vi "Main.vi"() -> ()   [LabVIEW 2019]
uses:
  _Sound/Music Player Command Message.ctl
  _Sound/Music Player Command.ctl
  <vilib>/numeric/Random Number (Range) DBL.vi
  <vilib>/numeric/Random Number (Range) U64.vi
  <vilib>/numeric/sub_Random U32.vi
  _Sound/Sound.lvlib
panel:
  in  "Enable Disasters":bool
  in  "Disaster Ring":u16(ring) caption="Disaster" items=["Earthquake", "Tornado", "UFO", "» Apocalypse «"]
  in  "Launch Disaster":bool
  in  "Enable Sounds":bool=TRUE
  in  "Random":bool
  out "Now Playing::":string
  in  "Enable Music":bool=TRUE
  in  "Random Disasters":bool
  out "LED Yellow Left":bool[](array[boolean])
  out "LED Yellow Right":bool[](array[boolean])
  out "LED Yellow Bottom":bool[](array[boolean])
  out "LED Yellow Top":bool[](array[boolean])
  out "LED Red Top":bool[](array[boolean])
  out "LED Red Right":bool[](array[boolean])
  out "LED Red Bottom":bool[](array[boolean])
  out "LED Red Left":bool[](array[boolean])
  out "Disasters":bool
  # "SimCity 2000\nToolkit for LabVIEW"
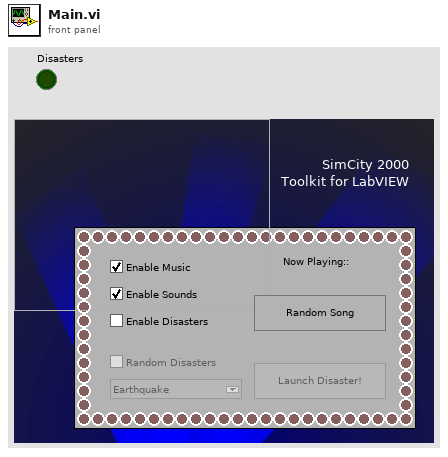
[diagram p1: front panel]
types:
  T1 = enum8{"Enabled", "Disabled", "Disabled and Grayed Out"}
  T2 = typedef "Sound.lvlib/Music Player Command Message.ctl" = cluster{"Command":T3, "Data":variant}
  T3 = typedef "Sound.lvlib/Music Player Command.ctl" = enum16{"Enable", "Play", "Play Random", "Stop", "Shutdown"}
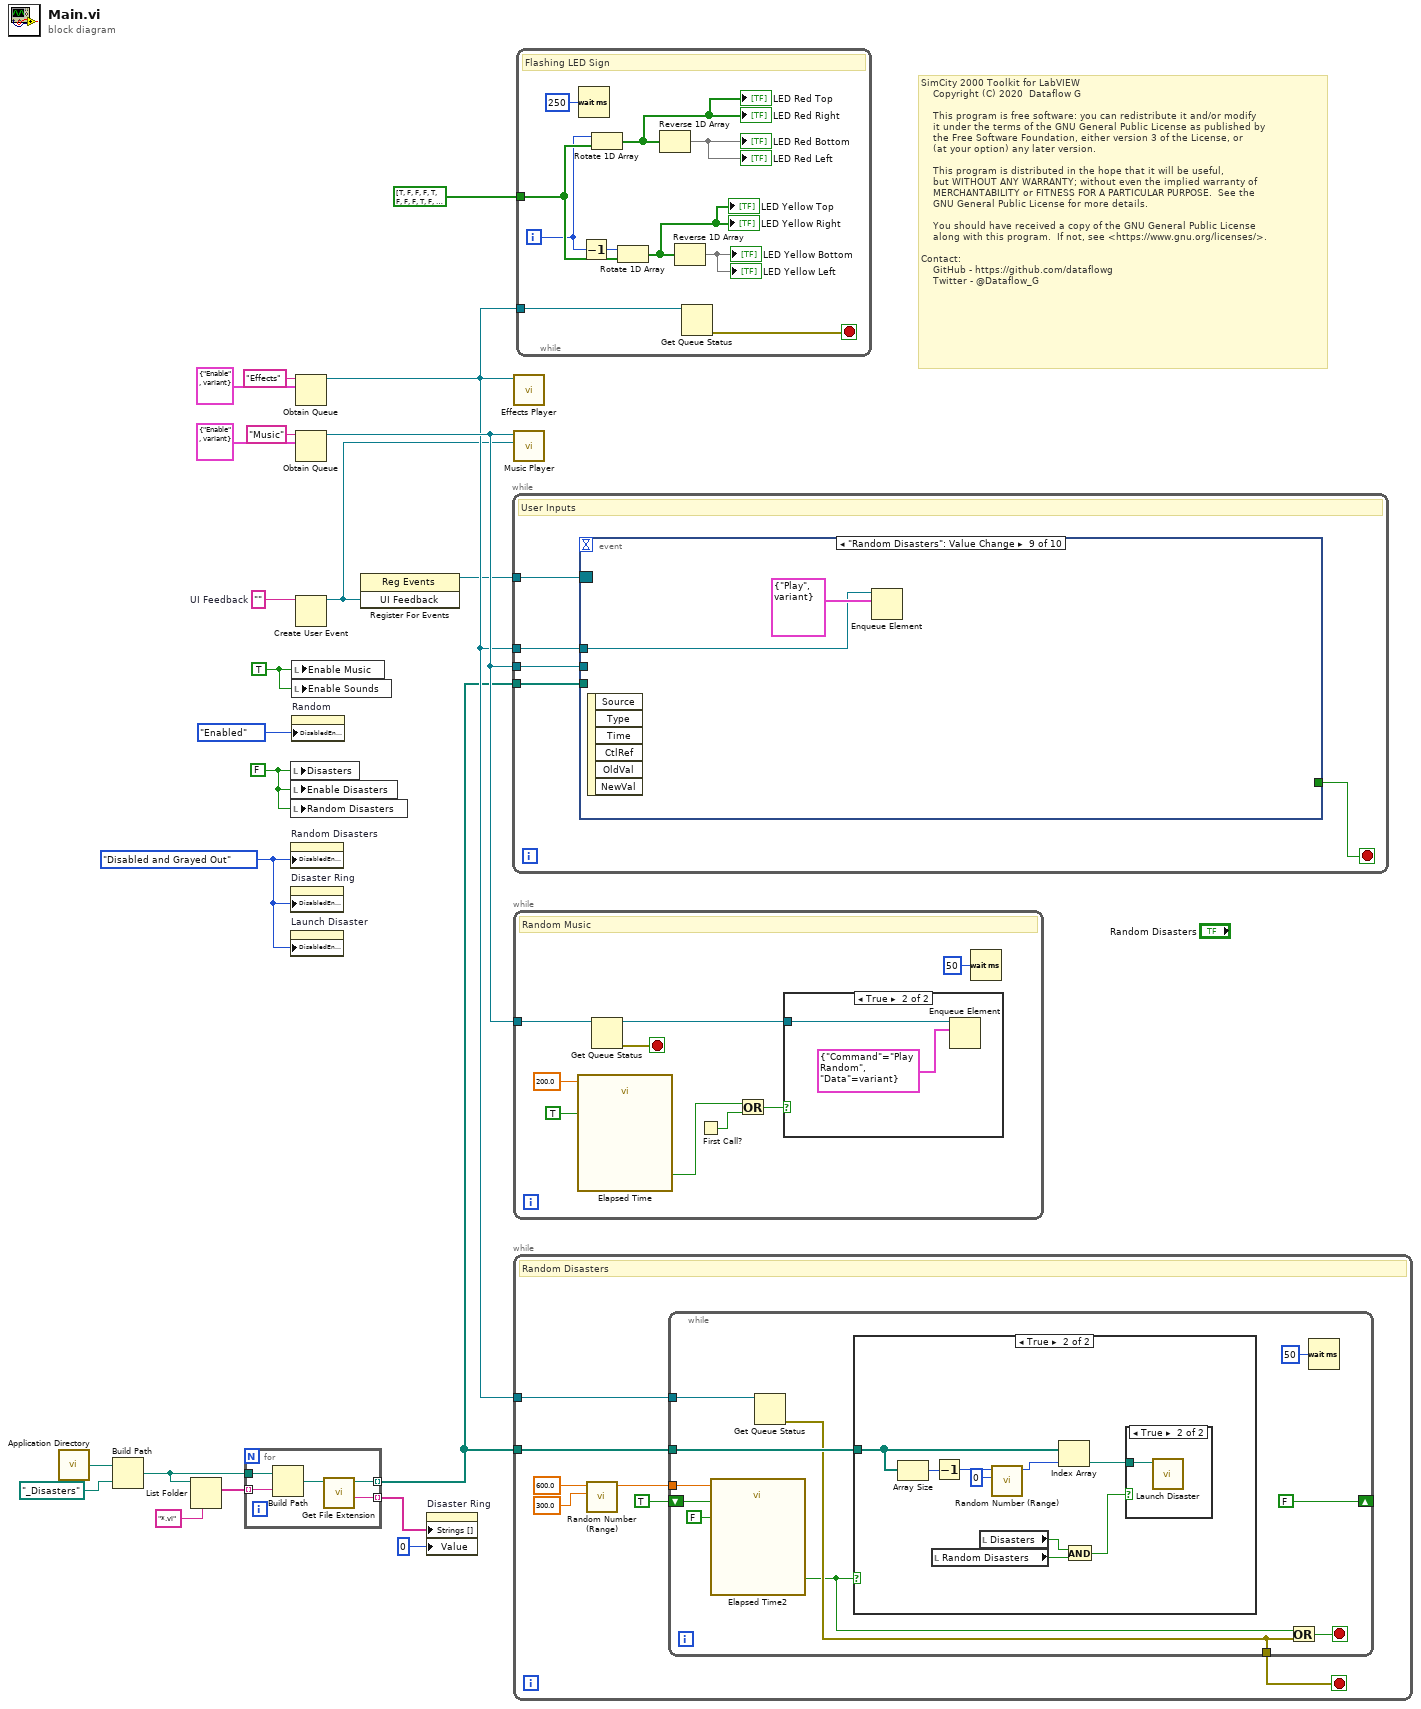
[diagram p0: block diagram]
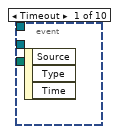
[diagram p5: hidden frame]
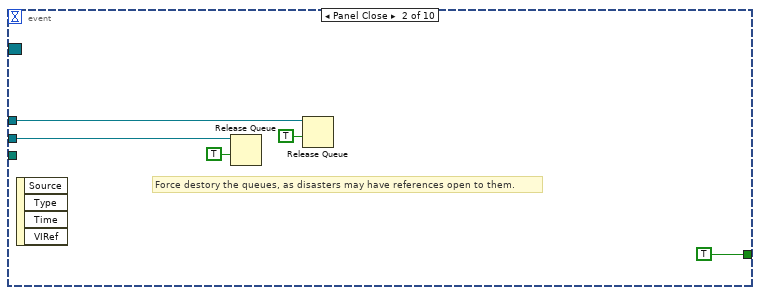
[diagram p6: hidden frame]
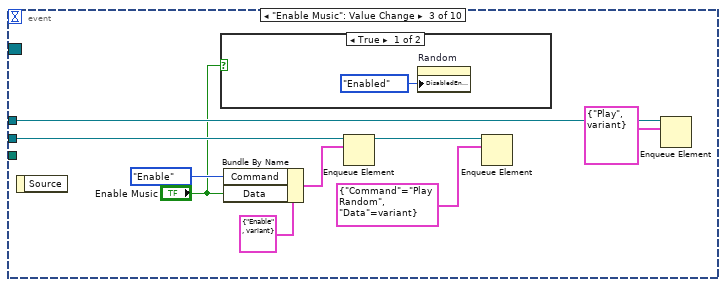
[diagram p7: hidden frame]
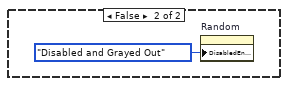
[diagram p8: hidden frame]
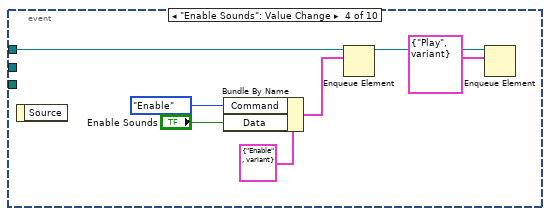
[diagram p9: hidden frame]
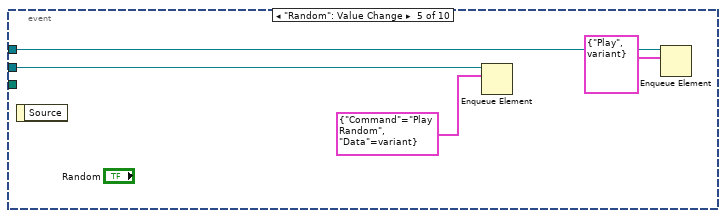
[diagram p10: hidden frame]
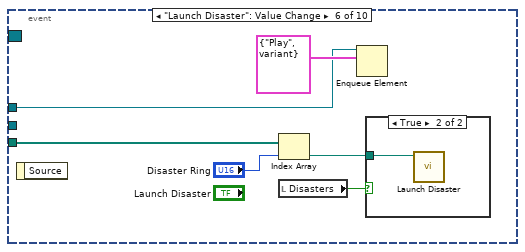
[diagram p11: hidden frame]
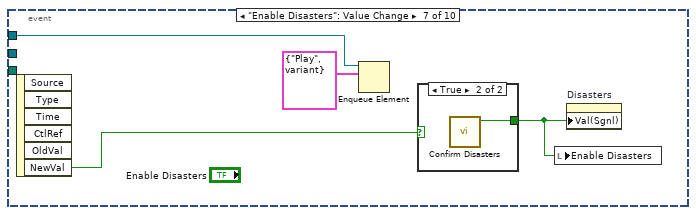
[diagram p13: hidden frame]
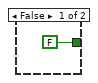
[diagram p14: hidden frame]
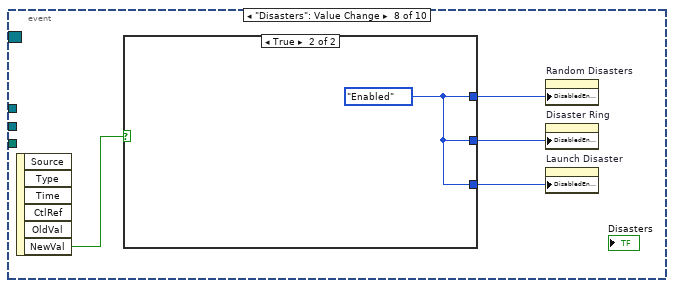
[diagram p15: hidden frame]
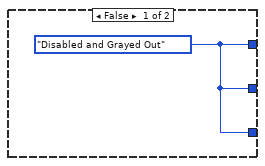
[diagram p16: hidden frame]
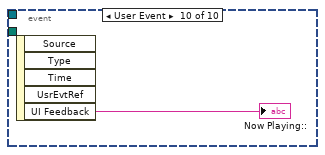
[diagram p17: hidden frame]
diagram:
  w1 = FALSE ("Disasters")
  w2 = TRUE ("Enable Music")
  w4 = T1."Disabled and Grayed Out" ("Disabled")
  w13 = ""  # UI Feedback
  # "SimCity 2000 Toolkit for LabVIEW\n    Copyright (C) 2020  Dataflow G\n    \n    This program is free software: you can redistribute it and/or modify\n    it under the terms of the GNU General Public License as published by\n    the Free Software Foundation, either version 3 of the License, or\n    (at your option) any later version.\n\n    This program is distributed in the hope that it will be useful,\n    but WITHOUT ANY WARRANTY; without even the implied warranty of\n    MERCHANTABILITY or FITNESS FOR A PARTICULAR PURPOSE.  See the\n    GNU General Public License for more details.\n\n    You should have received a copy of the GNU General Public License\n    along with this program.  If not, see <https://www.gnu.org/licenses/>.\n\nContact:\n    GitHub - https://github.com/dataflowg\n    Twitter - @Dataflow_G"
  n1 = call <vilib>:"Application Directory.vi"() -> ("Application Directory"=w20:path)
  n2 = Build Path(base path=w20, name or relative path=path "_Disasters" ("path")) -> (appended path=w10:path)
  n3 = List Folder(path=w10, pattern="*.vi") -> (filenames=w9:string[])  [unwired: 2 in, 3 out]
  n4 = for {
    tunnel: w10 -> [w27]
    tunnel: w9 -> [w26] mode=indexing
    tunnel: [w24] -> w7 mode=indexing
    tunnel: [w23] -> w5 mode=indexing
    n5 = Build Path(base path=w27, name or relative path=w26) -> (appended path=w25:path)
    n6 = call <vilib>:"Get File Extension.vi"("file"=w25) -> ("filename without extension"=w24:string, "dup file"=w23:path)  [unwired: 6 in, 3 out]
  }
  n7 = local write "Disasters"(w1) -> ()
  n8 = local write "Enable Disasters"(w1) -> ()
  n9 = local write "Random Disasters"(w1) -> ()
  n10 = property on="Random Disasters" class="Bool (strict)"("DisabledEnum"=w4) -> ()  [unwired: 2 in, 2 out]
  n11 = property on="Disaster Ring" class="Ring (strict)"("DisabledEnum"=w4) -> ()  [unwired: 2 in, 2 out]
  n12 = property on="Launch Disaster" class="Bool"("DisabledEnum"=w4) -> ()  [unwired: 2 in, 2 out]
  n13 = local write "Enable Music"(w2) -> ()
  n14 = local write "Enable Sounds"(w2) -> ()
  n15 = property on="Random" class="Bool"("DisabledEnum"=T1."Enabled" ("Disabled")) -> ()  [unwired: 2 in, 2 out]
  n16 = Obtain Queue(name (unnamed)="Effects", element data type=T2 {"Command"=enum."Enable", "Data"=variant} ("Message")) -> (queue out=w16:refnum<queue>)  [unwired: 3 in, 2 out]
  n17 = Obtain Queue(name (unnamed)="Music", element data type=T2 {"Command"=enum."Enable", "Data"=variant} ("Message")) -> (queue out=w19:refnum<queue>)  [unwired: 3 in, 2 out]
  n18 = Create User Event(user event datatype=w13) -> (user event=w12:refnum<user-event>)  [unwired: 1 in, 1 out]
  n19 = register-events(w12) -> (reference out=w11:refnum<event-registration>)  [unwired: 2 in, 1 out]
  n20 = property on="Disaster Ring" class="Ring (strict)"("Strings []"=w7, "Value"=u16 0) -> ()  [unwired: 2 in, 2 out]
  n21 = while {
    tunnel: w19 -> [w32]
    tunnel: w16 -> [w31]
    tunnel: w11 -> [w29]
    tunnel: w5 -> [w28]
    stop <- w30 stop-if-true
    # "User Inputs"
    n22 = event shown="[8] \"Random Disasters\": Value Change" {
      selector: w29 -> [_ _ _ _ _ _ _ _ _ _]
      dyn-events: _ -> [_ _ _ _ _ _ _ _ _ _]
      timeout: _ -> [_ _ _ _ _ _ _ _ _ _]
      tunnel: w32 -> [_ w37 w44 _ w56 _ _ _ _ _]
      tunnel: w31 -> [_ w36 w42 w50 w59 w60 w68 _ w79 _]
      tunnel: [_ TRUE _ _ _ _ _ _ _ _] -> w30
      tunnel: w28 -> [_ _ _ _ _ w65 _ _ _ _]
      event Timeout {
        n23 = event-data() -> ()  [unwired: 1 in, 3 out]
      }
      event Panel Close {
        # "Force destory the queues, as disasters may have references open to them."
        n24 = event-data() -> ()  [unwired: 1 in, 4 out]
        n25 = Release Queue(queue=w37, force destroy? (F)=TRUE) -> ()  [unwired: 1 in, 3 out]
        n26 = Release Queue(queue=w36, force destroy? (F)=TRUE) -> ()  [unwired: 1 in, 3 out]
      }
      event "Enable Music": Value Change {
        n27 = event-data() -> ()  [unwired: 1 in, 1 out]
        n28 = case shown="True" "Enable Music" {
          frame True {
            n29 = property on="Random" class="Bool"("DisabledEnum"=T1."Enabled" ("Disabled")) -> ()  [unwired: 2 in, 2 out]
          }
          frame False {
            n30 = property on="Random" class="Bool"("DisabledEnum"=T1."Disabled and Grayed Out" ("Disabled")) -> ()  [unwired: 2 in, 2 out]
          }
        }
        n31 = Bundle By Name(cluster=T2 {"Command"=enum."Enable", "Data"=variant} ("Message"), "Command"=Music_Player_Command."Enable", "Data"="Enable Music") -> (w43:T2)
        n32 = Enqueue Element(queue=w44, element=w43) -> (queue out=w40:refnum<queue>)  [unwired: 2 in, 2 out]
        n33 = Enqueue Element(queue=w40, element=T2 {"Command"=enum."Play Random", "Data"=variant} ("Message")) -> ()  [unwired: 2 in, 3 out]
        n34 = Enqueue Element(queue=w42, element=T2 {"Command"=enum."Play", "Data"=variant(string "click")}) -> ()  [unwired: 2 in, 3 out]
      }
      event "Enable Sounds": Value Change {
        n35 = event-data() -> ()  [unwired: 1 in, 1 out]
        n36 = Bundle By Name(cluster=T2 {"Command"=enum."Enable", "Data"=variant} ("Message"), "Command"=Music_Player_Command."Enable", "Data"="Enable Sounds") -> (w53:T2)
        n37 = Enqueue Element(queue=w50, element=w53) -> (queue out=w49:refnum<queue>)  [unwired: 2 in, 2 out]
        n38 = Enqueue Element(queue=w49, element=T2 {"Command"=enum."Play", "Data"=variant(string "click")}) -> ()  [unwired: 2 in, 3 out]
      }
      event "Random": Value Change {
        n39 = event-data() -> ()  [unwired: 1 in, 1 out]
        n40 = Enqueue Element(queue=w56, element=T2 {"Command"=enum."Play Random", "Data"=variant} ("Message")) -> ()  [unwired: 2 in, 3 out]
        n41 = Enqueue Element(queue=w59, element=T2 {"Command"=enum."Play", "Data"=variant(string "click")}) -> ()  [unwired: 2 in, 3 out]
      }
      event "Launch Disaster": Value Change {
        n42 = event-data() -> ()  [unwired: 1 in, 1 out]
        n43 = Index Array(array=w65, index="Disaster Ring") -> (element=w63:path)
        n44 = local read "Disasters"() -> (w62:bool)
        n45 = Enqueue Element(queue=w60, element=T2 {"Command"=enum."Play", "Data"=variant(string "click")}) -> ()  [unwired: 2 in, 3 out]
        n46 = case shown="True" w62 {
          tunnel: w63 -> [_ w66]
          frame False {
          }
          frame True {
            n47 = call "Launch Disaster.vi"("VI Path"=w66) -> ()  [unwired: 11 in]
          }
        }
      }
      event "Enable Disasters": Value Change {
        n48 = event-data() -> ("NewVal"=w70:bool)  [unwired: 1 in, 5 out]
        n49 = Enqueue Element(queue=w68, element=T2 {"Command"=enum."Play", "Data"=variant(string "click")}) -> ()  [unwired: 2 in, 3 out]
        n50 = case shown="True" w70 {
          tunnel: [FALSE ("T button?") w72] -> w67
          frame False {
          }
          frame True {
            n51 = call "Confirm Disasters.vi"() -> ("Enable Disasters"=w72:bool)  [unwired: 11 in]
          }
        }
        n52 = local write "Enable Disasters"(w67) -> ()
        n53 = property on="Disasters" class="Bool (strict)"("Val(Sgnl)"=w67) -> ()  [unwired: 2 in, 2 out]
      }
      event "Disasters": Value Change {
        n54 = event-data() -> ("NewVal"=w76:bool)  [unwired: 1 in, 5 out]
        n55 = case shown="True" w76 {
          tunnel: [w77 w78] -> w75
          tunnel: [w77 w78] -> w74
          tunnel: [w77 w78] -> w73
          frame False {
            w77 = T1."Disabled and Grayed Out" ("Disabled")
          }
          frame True {
            w78 = T1."Enabled" ("Disabled")
          }
        }
        n56 = property on="Random Disasters" class="Bool (strict)"("DisabledEnum"=w75) -> ()  [unwired: 2 in, 2 out]
        n57 = property on="Disaster Ring" class="Ring (strict)"("DisabledEnum"=w74) -> ()  [unwired: 2 in, 2 out]
        n58 = property on="Launch Disaster" class="Bool"("DisabledEnum"=w73) -> ()  [unwired: 2 in, 2 out]
      }
      event "Random Disasters": Value Change {
        n59 = event-data() -> ()  [unwired: 1 in, 6 out]
        n60 = Enqueue Element(queue=w79, element=T2 {"Command"=enum."Play", "Data"=variant(string "click")}) -> ()  [unwired: 2 in, 3 out]
      }
      event User Event {
        n61 = event-data() -> ("UI Feedback"=→"Now Playing::":string)  [unwired: 1 in, 4 out]
      }
    }
  }
  n62 = call "Effects Player.vi"("Command Queue"=w16) -> ()  [unwired: 11 in]
  n63 = call "Music Player.vi"("UI Feedback"=w12, "Command Queue"=w19) -> ()  [unwired: 10 in]
  n64 = while {
    tunnel: w19 -> [w83]
    stop <- w82 stop-if-true
    # "Random Music"
    n65 = call "Elapsed Time"("Time Target (s)"=200.0, "Auto Reset"=TRUE) -> ("Time has Elapsed"=w88:bool)  [unwired: 10 in, 7 out]
    n66 = Get Queue Status(queue=w83) -> (queue out=w84:refnum<queue>, error out=w82:errorcluster)  [unwired: 2 in, 6 out]
    n67 = First Call?() -> (First Call?: T/F=w89:bool)
    n68 = Or(x=w88, y=w89) -> (x .or. y?=w87:bool)
    n69 = case shown="True" w87 {
      tunnel: w84 -> [_ w92]
      frame False {
      }
      frame True {
        n70 = Enqueue Element(queue=w92, element=T2 {"Command"=enum."Play Random", "Data"=variant} ("Message")) -> ()  [unwired: 2 in, 3 out]
      }
    }
    n71 = Wait (ms)(milliseconds to wait=u32 50) -> ()  [unwired: 1 out]
  }
  n72 = while {
    tunnel: w5 -> [w99]
    tunnel: w16 -> [w95]
    stop <- w94 stop-if-true
    # "Random Disasters"
    n73 = call-poly <vilib>:"Random Number (Range).vi"("lower bound (0)"=300.0, "upper bound (100)"=600.0) -> ("number"=w93:dbl)  [unwired: 9 in]
    n74 = while {
      tunnel: w99 -> [w109]
      tunnel: w93 -> [w108]
      shift-right: [FALSE ("Reset")] -> _
      shift-left: TRUE ("Reset") -> [w106]
      tunnel: w95 -> [w103]
      tunnel: [w101] -> w94
      stop <- w102 stop-if-true
      n75 = call "Elapsed Time2"("Time Target (s)"=w108, "Reset"=w106, "Auto Reset"=FALSE) -> ("Time has Elapsed"=w100:bool)  [unwired: 9 in, 7 out]
      n76 = Get Queue Status(queue=w103) -> (error out=w101:errorcluster)  [unwired: 2 in, 7 out]
      n77 = case shown="True" w100 {
        tunnel: w109 -> [_ w117]
        frame False {
        }
        frame True {
          n78 = Array Size(array=w117) -> (size(s)=w116:i32)
          n79 = local read "Random Disasters"() -> (w111:bool)
          n80 = Decrement(x=w116) -> (x-1=w114:i32)
          n81 = local read "Disasters"() -> (w112:bool)
          n82 = call-poly <vilib>:"Random Number (Range).vi"("lower bound (0)"=u64 0, "upper bound (100)"=w114) -> ("number"=w113:u64)  [unwired: 9 in]
          n83 = Index Array(array=w117, index=w113) -> (element=w118:path)
          n84 = And(x=w112, y=w111) -> (x .and. y?=w110:bool)
          n85 = case shown="True" w110 {
            tunnel: w118 -> [_ w119]
            frame False {
            }
            frame True {
              n86 = call "Launch Disaster.vi"("VI Path"=w119) -> ()  [unwired: 11 in]
            }
          }
        }
      }
      n87 = Or(x=w100, y=w101) -> (x .or. y?=w102:bool)
      n88 = Wait (ms)(milliseconds to wait=u32 50) -> ()  [unwired: 1 out]
    }
  }
  n89 = while {
    tunnel: bool[] [TRUE, FALSE, FALSE, FALSE, TRUE, FALSE, FALSE, FALSE, TRUE, FALSE, FALSE, FALSE, TRUE, FALSE, FALSE, FALSE, TRUE, FALSE, FALSE, FALSE, TRUE, FALSE, FALSE, FALSE, TRUE, FALSE, FALSE, FALSE, TRUE, FALSE, FALSE, FALSE] ("Array") -> [w127]
    tunnel: w16 -> [w121]
    i -> [w126]
    stop <- w120 stop-if-true
    # "Flashing LED Sign"
    n90 = Wait (ms)(milliseconds to wait=u32 250) -> ()  [unwired: 1 out]
    n91 = Decrement(x=w126) -> (x-1=w125:i32)
    n92 = Rotate 1D Array(1:w127, 2:w126) -> (0:w124:bool[])
    "LED Red Top" <- w124
    "LED Red Right" <- w124
    n93 = Rotate 1D Array(1:w127, 2:w125) -> (0:w123:bool[])
    "LED Yellow Top" <- w123
    "LED Yellow Right" <- w123
    n94 = Reverse 1D Array(array=w124) -> (reversed array=→"LED Red Bottom" →"LED Red Left":bool[])
    n95 = Reverse 1D Array(array=w123) -> (reversed array=→"LED Yellow Left" →"LED Yellow Bottom":bool[])
    n96 = Get Queue Status(queue=w121) -> (error out=w120:errorcluster)  [unwired: 2 in, 7 out]
  }
